vi "Game_of_Life.vi"() -> ()   [LabVIEW 2018]
panel:
  in  "Probability of \nRandom Generation (％)":dbl=30.0
  in  "Time Interval (ms)":u32=500
  in  "Size of Grid":i32=20
  in  "Random Generation":bool
  in  "Reset":bool
  in  "Start":bool
  in  "Stop":bool
  in  "Cells":bool[][](array[boolean])
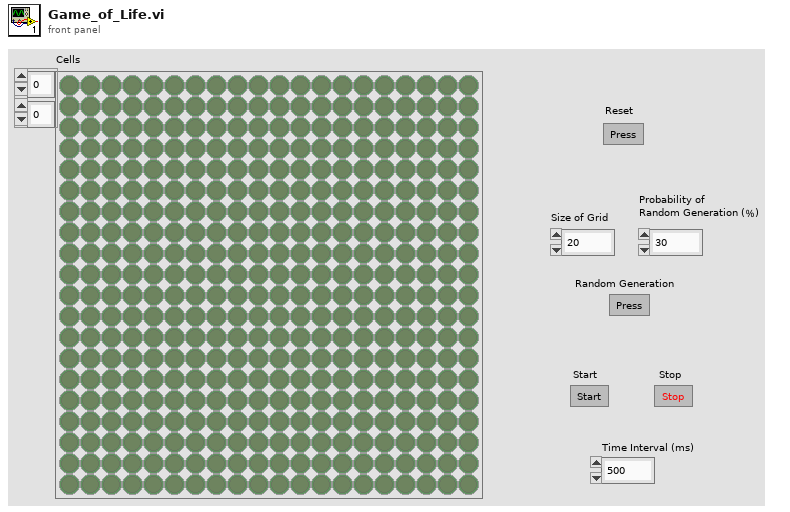
[diagram p1: front panel]
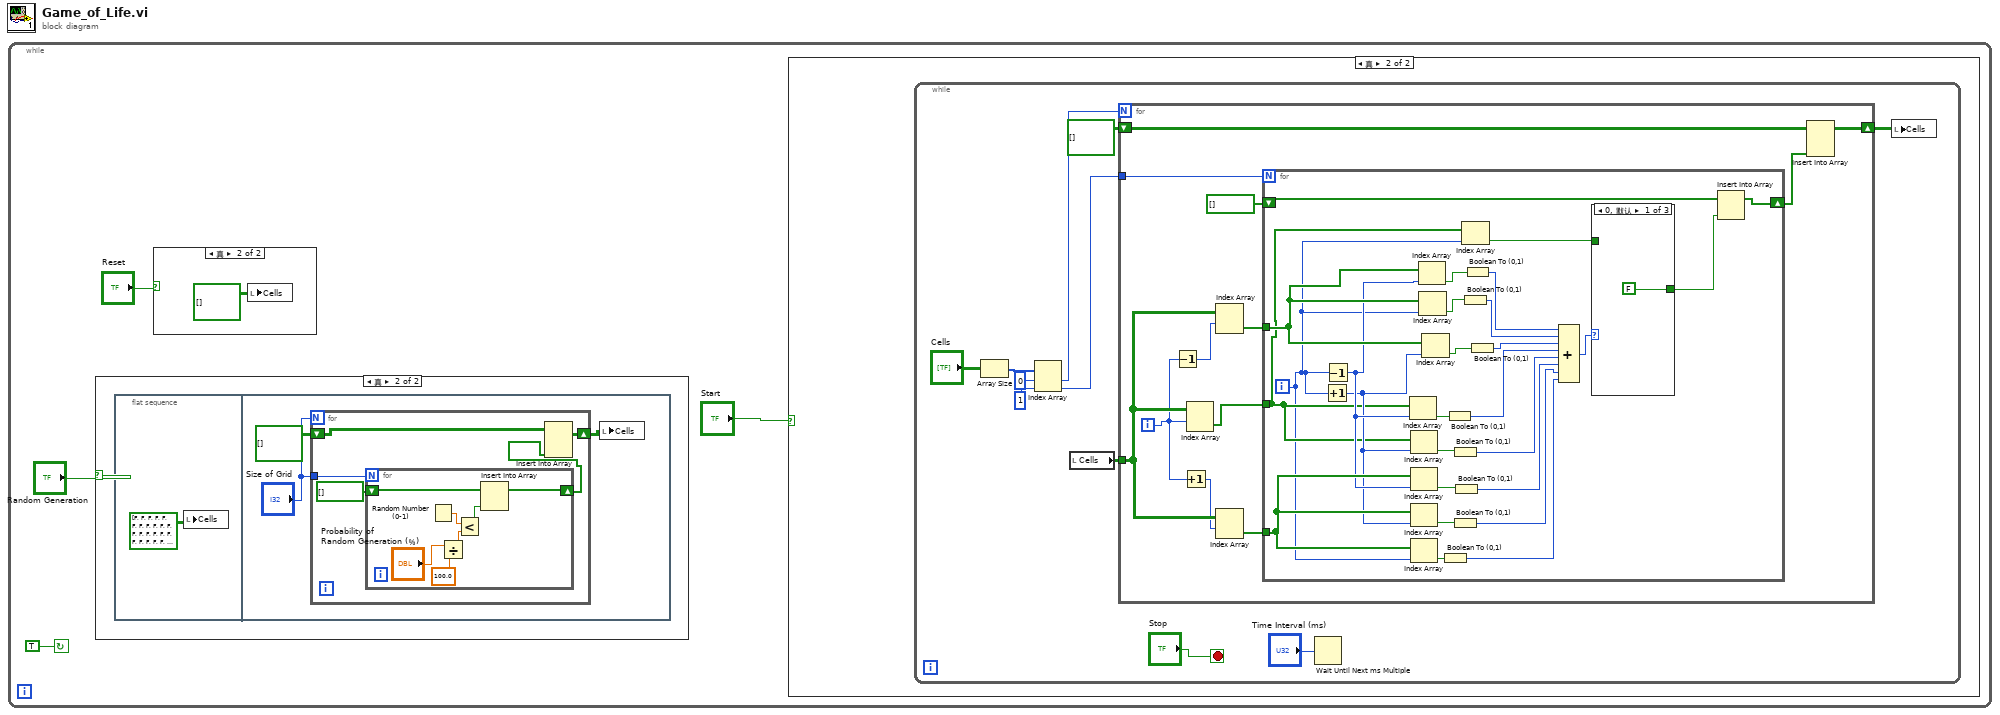
[diagram p0: block diagram]
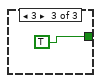
[diagram p4: hidden frame]
diagram:
  n1 = while {
    stop <- TRUE continue-if-true
    n2 = case shown="真" "Random Generation" {
      frame False {
      }
      frame True {
        n3 = flat-sequence {
          frame #0 {
            n4 = local write "Cells"(bool[][] [[FALSE, FALSE, FALSE, FALSE, FALSE, FALSE, FALSE, FALSE, FALSE, FALSE, FALSE, FALSE, FALSE, FALSE, FALSE, FALSE, FALSE, FALSE, FALSE, FALSE], [FALSE, FALSE, FALSE, FALSE, FALSE, FALSE, FALSE, FALSE, FALSE, FALSE, FALSE, FALSE, FALSE, FALSE, FALSE, FALSE, FALSE, FALSE, FALSE, FALSE], [FALSE, FALSE, FALSE, FALSE, FALSE, FALSE, FALSE, FALSE, FALSE, FALSE, FALSE, FALSE, FALSE, FALSE, FALSE, FALSE, FALSE, FALSE, FALSE, FALSE], [FALSE, FALSE, FALSE, FALSE, FALSE, FALSE, FALSE, FALSE, FALSE, FALSE, FALSE, FALSE, FALSE, FALSE, FALSE, FALSE, FALSE, FALSE, FALSE, FALSE], [FALSE, FALSE, FALSE, FALSE, FALSE, FALSE, FALSE, FALSE, FALSE, FALSE, FALSE, FALSE, FALSE, FALSE, FALSE, FALSE, FALSE, FALSE, FALSE, FALSE], [FALSE, FALSE, FALSE, FALSE, FALSE, FALSE, FALSE, FALSE, FALSE, FALSE, FALSE, FALSE, FALSE, FALSE, FALSE, FALSE, FALSE, FALSE, FALSE, FALSE], [FALSE, FALSE, FALSE, FALSE, FALSE, FALSE, FALSE, FALSE, FALSE, FALSE, FALSE, FALSE, FALSE, FALSE, FALSE, FALSE, FALSE, FALSE, FALSE, FALSE], [FALSE, FALSE, FALSE, FALSE, FALSE, FALSE, FALSE, FALSE, FALSE, FALSE, FALSE, FALSE, FALSE, FALSE, FALSE, FALSE, FALSE, FALSE, FALSE, FALSE], [FALSE, FALSE, FALSE, FALSE, FALSE, FALSE, FALSE, FALSE, FALSE, FALSE, FALSE, FALSE, FALSE, FALSE, FALSE, FALSE, FALSE, FALSE, FALSE, FALSE], [FALSE, FALSE, FALSE, FALSE, FALSE, FALSE, FALSE, FALSE, FALSE, FALSE, FALSE, FALSE, FALSE, FALSE, FALSE, FALSE, FALSE, FALSE, FALSE, FALSE], [FALSE, FALSE, FALSE, FALSE, FALSE, FALSE, FALSE, FALSE, FALSE, FALSE, FALSE, FALSE, FALSE, FALSE, FALSE, FALSE, FALSE, FALSE, FALSE, FALSE], [FALSE, FALSE, FALSE, FALSE, FALSE, FALSE, FALSE, FALSE, FALSE, FALSE, FALSE, FALSE, FALSE, FALSE, FALSE, FALSE, FALSE, FALSE, FALSE, FALSE], [FALSE, FALSE, FALSE, FALSE, FALSE, FALSE, FALSE, FALSE, FALSE, FALSE, FALSE, FALSE, FALSE, FALSE, FALSE, FALSE, FALSE, FALSE, FALSE, FALSE], [FALSE, FALSE, FALSE, FALSE, FALSE, FALSE, FALSE, FALSE, FALSE, FALSE, FALSE, FALSE, FALSE, FALSE, FALSE, FALSE, FALSE, FALSE, FALSE, FALSE], [FALSE, FALSE, FALSE, FALSE, FALSE, FALSE, FALSE, FALSE, FALSE, FALSE, FALSE, FALSE, FALSE, FALSE, FALSE, FALSE, FALSE, FALSE, FALSE, FALSE], [FALSE, FALSE, FALSE, FALSE, FALSE, FALSE, FALSE, FALSE, FALSE, FALSE, FALSE, FALSE, FALSE, FALSE, FALSE, FALSE, FALSE, FALSE, FALSE, FALSE], [FALSE, FALSE, FALSE, FALSE, FALSE, FALSE, FALSE, FALSE, FALSE, FALSE, FALSE, FALSE, FALSE, FALSE, FALSE, FALSE, FALSE, FALSE, FALSE, FALSE], [FALSE, FALSE, FALSE, FALSE, FALSE, FALSE, FALSE, FALSE, FALSE, FALSE, FALSE, FALSE, FALSE, FALSE, FALSE, FALSE, FALSE, FALSE, FALSE, FALSE], [FALSE, FALSE, FALSE, FALSE, FALSE, FALSE, FALSE, FALSE, FALSE, FALSE, FALSE, FALSE, FALSE, FALSE, FALSE, FALSE, FALSE, FALSE, FALSE, FALSE], [FALSE, FALSE, FALSE, FALSE, FALSE, FALSE, FALSE, FALSE, FALSE, FALSE, FALSE, FALSE, FALSE, FALSE, FALSE, FALSE, FALSE, FALSE, FALSE, FALSE]] ("数组")) -> ()
          }
          frame #1 {
            n5 = for {
              N: "Size of Grid" -> [_]
              tunnel: "Size of Grid" -> [w67]
              shift-right: [w65] -> w61
              shift-left: bool[][] [] -> [w63]
              n6 = for {
                N: w67 -> [_]
                shift-right: [w73] -> w64
                shift-left: bool[] [] -> [w74]
                n7 = Random Number (0-1)() -> (number: 0 to 1=w70:dbl)
                n8 = Divide(x="Probability of \nRandom Generation (％)", y=100.0) -> (x/y=w69:dbl)
                n9 = Less?(x=w70, y=w69) -> (x < y?=w68:bool)
                n10 = Insert Into Array(array=w74, new element=w68) -> (w73:bool[])  [unwired: 1 in]
              }
              n11 = Insert Into Array(array=w63, new element=w64) -> (w65:bool[][])  [unwired: 2 in]
            }
            n12 = local write "Cells"(w61) -> ()
          }
        }
      }
    }
    n13 = case shown="真" "Reset" {
      frame False {
      }
      frame True {
        n14 = local write "Cells"(bool[][] [] ("数组")) -> ()
      }
    }
    n15 = case shown="真" "Start" {
      frame False {
      }
      frame True {
        n16 = while {
          stop <- "Stop" stop-if-true
          n17 = Array Size(array="Cells") -> (size(s)=w9:i32[])
          n18 = Index Array(array=w9, index #1=0 ("索引"), index #2=1 ("索引")) -> (element #1=w6:i32, element #2=w5:i32)
          n19 = local read "Cells"() -> (w13:bool[][])
          n20 = for {
            N: w6 -> [_]
            tunnel: w13 -> [w27]
            shift-right: [w18] -> w11
            shift-left: bool[][] [] -> [w17]
            tunnel: w5 -> [w16]
            i -> [w25]
            n21 = Decrement(x=w25) -> (x-1=w26:i32)
            n22 = Increment(x=w25) -> (x+1=w24:i32)
            n23 = Index Array(array=w27, index (row)=w25) -> (element=w22:bool[])  [unwired: 1 in]
            n24 = Index Array(array=w27, index (row)=w26) -> (element=w23:bool[])  [unwired: 1 in]
            n25 = Index Array(array=w27, index (row)=w24) -> (element=w21:bool[])  [unwired: 1 in]
            n26 = for {
              N: w16 -> [_]
              tunnel: w23 -> [w54]
              tunnel: w22 -> [w33]
              tunnel: w21 -> [w53]
              shift-right: [w28] -> w19
              shift-left: bool[] [] -> [w29]
              i -> [w32]
              n27 = Increment(x=w32) -> (x+1=w51:i32)
              n28 = Decrement(x=w32) -> (x-1=w52:i32)
              n29 = Index Array(array=w33, index=w52) -> (element=w49:bool)
              n30 = Index Array(array=w33, index=w51) -> (element=w48:bool)
              n31 = Index Array(array=w53, index=w52) -> (element=w47:bool)
              n32 = Index Array(array=w53, index=w51) -> (element=w46:bool)
              n33 = Index Array(array=w53, index=w32) -> (element=w45:bool)
              n34 = Index Array(array=w54, index=w52) -> (element=w43:bool)
              n35 = Index Array(array=w54, index=w32) -> (element=w44:bool)
              n36 = Index Array(array=w54, index=w51) -> (element=w50:bool)
              n37 = Boolean To (0,1)(Boolean=w45) -> (0, 1=w39:i16)
              n38 = Boolean To (0,1)(Boolean=w49) -> (0, 1=w35:i16)
              n39 = Boolean To (0,1)(Boolean=w48) -> (0, 1=w36:i16)
              n40 = Boolean To (0,1)(Boolean=w46) -> (0, 1=w38:i16)
              n41 = Boolean To (0,1)(Boolean=w47) -> (0, 1=w37:i16)
              n42 = Boolean To (0,1)(Boolean=w44) -> (0, 1=w41:i16)
              n43 = Index Array(array=w33, index=w32) -> (element=w30:bool)
              n44 = Boolean To (0,1)(Boolean=w43) -> (0, 1=w42:i16)
              n45 = Boolean To (0,1)(Boolean=w50) -> (0, 1=w40:i16)
              n46 = Compound Arithmetic op=ADD(w42, w41, w40, w35, w36, w37, w38, w39) -> (w34:i16)
              n47 = case shown="0, 默认" w34 {
                tunnel: [FALSE w56 TRUE] -> w31
                tunnel: w30 -> [_ w56 _]
                frame 0, Default {
                }
                frame 2 {
                }
                frame 3 {
                }
              }
              n48 = Insert Into Array(array=w29, new element=w31) -> (w28:bool[])  [unwired: 1 in]
            }
            n49 = Insert Into Array(array=w17, new element=w19) -> (w18:bool[][])  [unwired: 2 in]
          }
          n50 = Wait Until Next ms Multiple(millisecond multiple="Time Interval (ms)") -> ()  [unwired: 1 out]
          n51 = local write "Cells"(w11) -> ()
        }
      }
    }
  }
